vi "From Serial Form.vi"(6 "Serial Version":T1, 10 "Deserializer in":refnum<class "Deserializer.lvclass">, 11 "PAS Data in":refnum<class "PAS Data.lvclass">) -> (0 "error out":errorcluster, 2 "Deserializer out":refnum<class "Deserializer.lvclass">, 3 "PAS Data out":refnum<class "PAS Data.lvclass">)   [LabVIEW 2014, in "PAS Data.lvclass"]
uses:
  PAS Data.lvclass
  <vilib>/NI/AQ Character Lineator/Deserializer/Deserializer.lvclass
  <vilib>/NI/AQ Character Lineator/Serialization Common/Serial Version.ctl
  Cell/PAS Cell Data.lvclass
  PAS Data.lvclass/PAS Data.ctl
  <vilib>/NI/AQ Character Lineator/Serializable/Remove Timestamp.vi
  <vilib>/NI/AQ Character Lineator/Serializable/Remove Boolean.vi
  <vilib>/NI/AQ Character Lineator/Serializable/Remove Serializable Array.vi
  Data/Data.lvclass
  <vilib>/NI/AQ Character Lineator/Serializable/Serializable.lvclass
  <vilib>/NI/AQ Character Lineator/Serialization Common/Serialization Common.lvlib
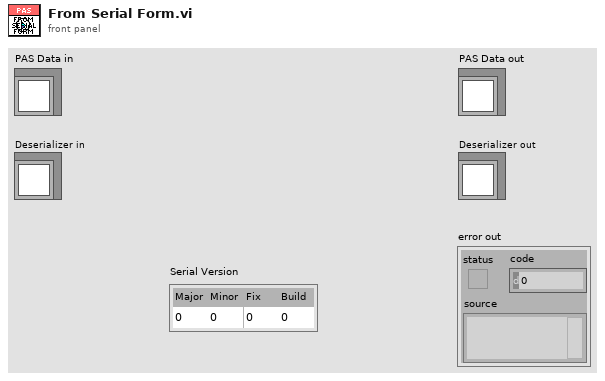
[diagram p1: front panel]
types:
  T1 = typedef "Serialization Common.lvlib/Serial Version.ctl" = cluster{"Major":u16, "Minor":u16, "Fix":u16, "Build":u16}
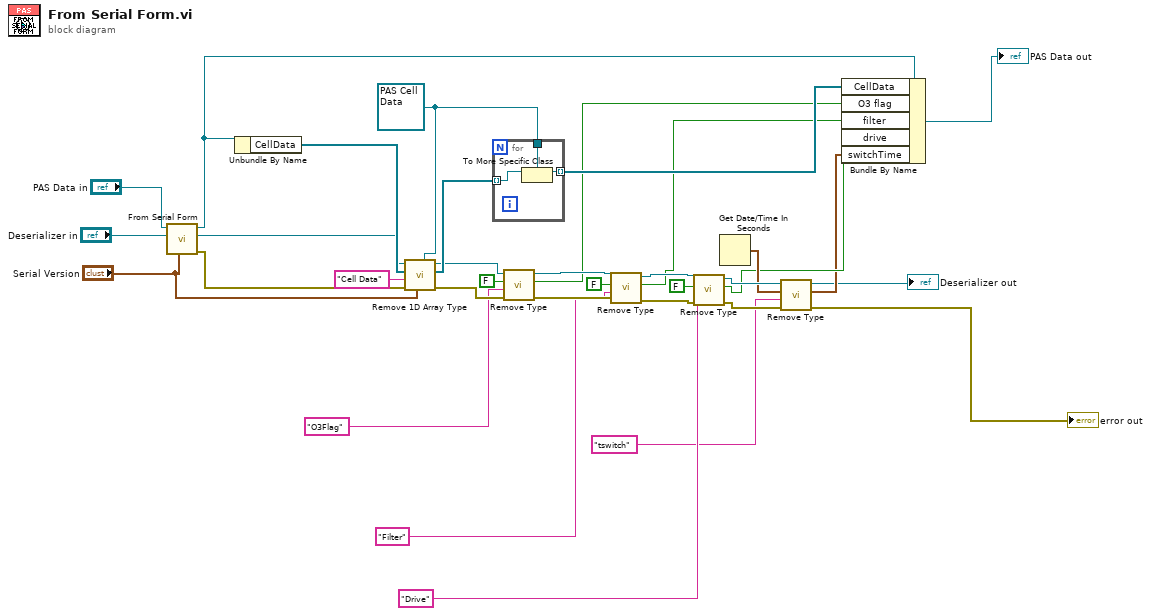
[diagram p0: block diagram]
diagram:
  w24 = refnum<class "PAS Cell Data.lvclass"> refnum ("PAS Cell Data.lvclass")
  n1 = call-parent "From Serial Form.vi"("Serial Version"="Serial Version", "Deserializer in"="Deserializer in", "Data in"="PAS Data in") -> ("error out"=w30:errorcluster, "Deserializer out"=w31:refnum<class "Deserializer.lvclass">, "Data out"=w9:refnum<class "PAS Data.lvclass">)  [unwired: 6 in]
  n2 = Unbundle By Name(w9) -> ("CellData"=w32:refnum<class "PAS Cell Data.lvclass">[])
  n3 = call-poly <vilib>:"Remove 1D Array Type.vi"("Default Serializable Type"=w24, "Serial Version"="Serial Version", "error in (no error)"=w30, "Name"="Cell Data", "Default Value"=w32, "Deserializer in"=w31) -> ("error out"=w26:errorcluster, "Serializables"=w27:refnum<class "Serializable.lvclass">[], "Deserializer out"=w25:refnum<class "Deserializer.lvclass">)  [unwired: 2 in, 1 out]
  n4 = for {
    tunnel: w27 -> [w37] mode=indexing
    tunnel: w24 -> [w36]
    tunnel: [w35] -> w8 mode=indexing
    n5 = To More Specific Class(target class=w36, reference=w37) -> (specific class reference=w35:refnum<class "PAS Cell Data.lvclass">)  [unwired: 1 in, 1 out]
  }
  n6 = call-poly <vilib>:"Remove Type.vi"("error in (no error)"=w26, "Name"="O3Flag", "Default Value"=FALSE, "Deserializer in"=w25) -> ("error out"=w19:errorcluster, "Boolean"=w7:bool, "Deserializer out"=w20:refnum<class "Deserializer.lvclass">)  [unwired: 4 in, 1 out]
  n7 = call-poly <vilib>:"Remove Type.vi"("error in (no error)"=w19, "Name"="Filter", "Default Value"=FALSE, "Deserializer in"=w20) -> ("error out"=w15:errorcluster, "Boolean"=w6:bool, "Deserializer out"=w16:refnum<class "Deserializer.lvclass">)  [unwired: 4 in, 1 out]
  n8 = call-poly <vilib>:"Remove Type.vi"("error in (no error)"=w15, "Name"="Drive", "Default Value"=FALSE, "Deserializer in"=w16) -> ("error out"=w12:errorcluster, "Boolean"=w5:bool, "Deserializer out"=w13:refnum<class "Deserializer.lvclass">)  [unwired: 4 in, 1 out]
  n9 = Get Date/Time In Seconds() -> (seconds since 1Jan1904=w11:timestamp)
  n10 = call-poly <vilib>:"Remove Type.vi"("error in (no error)"=w12, "Name"="tswitch", "Default Value"=w11, "Deserializer in"=w13) -> ("error out"=→"error out":errorcluster, "Time Stamp"=w4:timestamp, "Deserializer out"=→"Deserializer out":refnum<class "Deserializer.lvclass">)  [unwired: 4 in, 1 out]
  n11 = Bundle By Name(cluster=w9, "CellData"=w8, "O3 flag"=w7, "filter"=w6, "drive"=w5, "switchTime"=w4) -> (→"PAS Data out":refnum<class "PAS Data.lvclass">)
